vi "email_alert.vi"(6 "Email Alert - Message":string, 9 "Email Alert - Engineer":string, 10 "Email Alert - CC":string, 11 "Email ALert - Attachment":path) -> ()   [LabVIEW 2011]
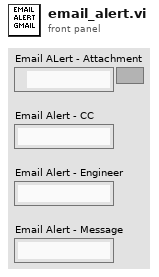
[diagram p1: front panel]
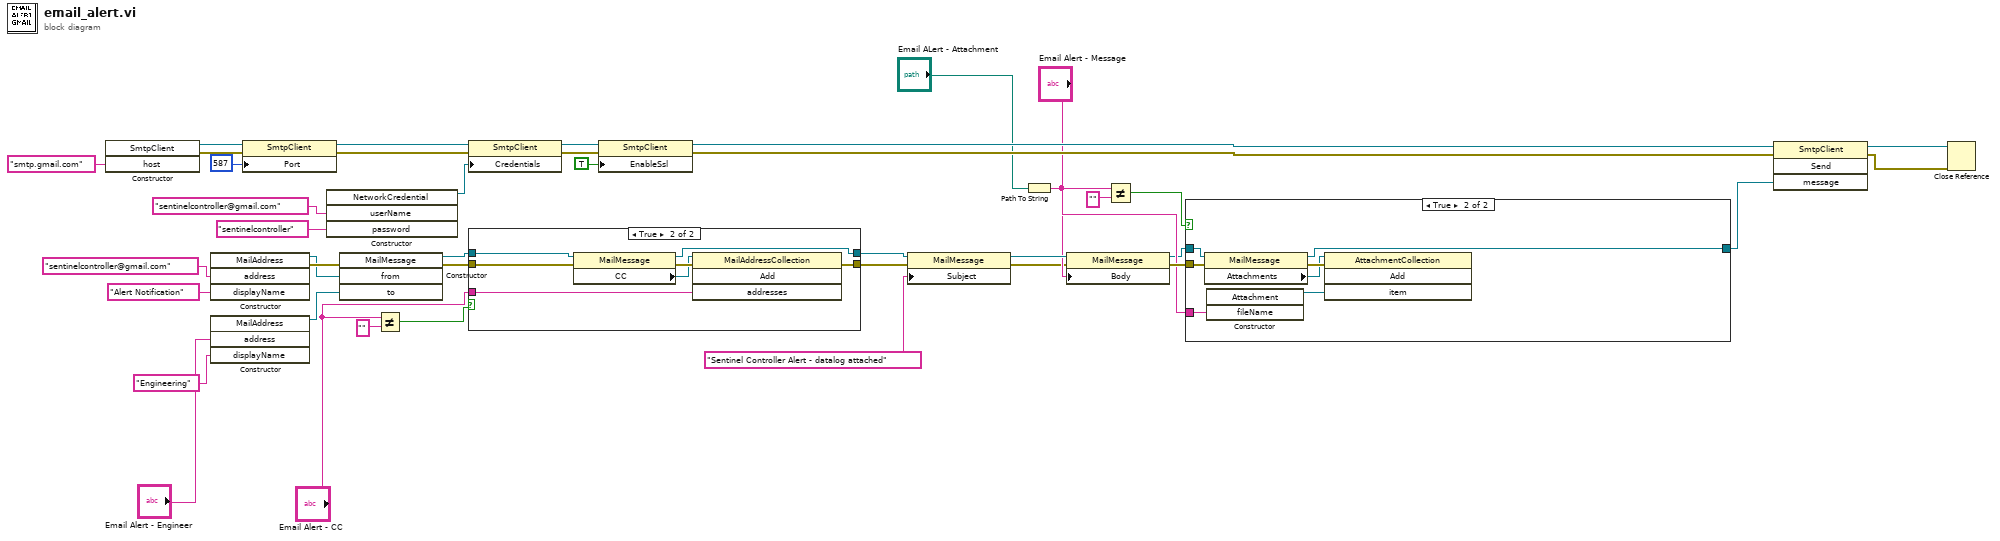
[diagram p0: block diagram]
diagram:
  n1 = constructor class="SmtpClient"("host"="smtp.gmail.com") -> (reference out=w10:refnum<k24>, error out=w13:errorcluster)  [unwired: 3 in, 2 out]
  n2 = constructor class="MailAddress"("address"="sentinelcontroller@gmail.com", "displayName"="Alert Notification") -> (reference out=w4:refnum<k24>, error out=w31:errorcluster)  [unwired: 3 in, 3 out]
  n3 = constructor class="MailAddress"("address"="Email Alert - Engineer", "displayName"="Engineering") -> (reference out=w3:refnum<k24>)  [unwired: 3 in, 4 out]
  n4 = property class="SmtpClient"(reference=w10, error in=w13, "Port"=587) -> (reference out=w11:refnum<k24>, error out=w14:errorcluster)
  n5 = constructor class="NetworkCredential"("userName"="sentinelcontroller@gmail.com", "password"="sentinelcontroller") -> (reference out=w9:refnum<k24>)  [unwired: 3 in, 4 out]
  n6 = constructor class="MailMessage"(error in=w31, "from"=w4, "to"=w3) -> (reference out=w24:refnum<k24>, error out=w25:errorcluster)  [unwired: 2 in, 3 out]
  n7 = Not Equal?(x="Email Alert - CC", y="") -> (x != y?=w22:bool)
  n8 = property class="SmtpClient"(reference=w11, error in=w14, "Credentials"=w9) -> (reference out=w12:refnum<k24>, error out=w15:errorcluster)
  n9 = case shown="True" w22 {
    tunnel: "Email Alert - CC" -> [_ w48]
    tunnel: w24 -> [w43 w47]
    tunnel: w25 -> [w42 w46]
    tunnel: [w43 w45] -> w26
    tunnel: [w42 w44] -> w27
    frame False {
    }
    frame True {
      n10 = property class="MailMessage"(reference=w47, error in=w46) -> (reference out=w45:refnum<k24>, error out=w50:errorcluster, "CC"=w49:refnum<k24>)
      n11 = invoke class="MailAddressCollection" method="Add"(reference=w49, error in=w50, "addresses"=w48) -> (error out=w44:errorcluster)  [unwired: 1 in, 3 out]
    }
  }
  n12 = property class="SmtpClient"(reference=w12, error in=w15, "EnableSsl"=TRUE) -> (reference out=w30:refnum<k24>, error out=w29:errorcluster)
  n13 = property class="MailMessage"(reference=w26, error in=w27, "Subject"="Sentinel Controller Alert - datalog attached") -> (reference out=w8:refnum<k24>, error out=w5:errorcluster)
  n14 = Path To String(path="Email ALert - Attachment") -> (string=w20:string)
  n15 = property class="MailMessage"(reference=w8, error in=w5, "Body"="Email Alert - Message") -> (reference out=w16:refnum<k24>, error out=w32:errorcluster)
  n16 = Not Equal?(x=w20, y="") -> (x != y?=w19:bool)
  n17 = case shown="True" w19 {
    tunnel: w16 -> [w51 w55]
    tunnel: [w51 w54] -> w28
    tunnel: w20 -> [_ w53]
    tunnel: w32 -> [_ w52]
    frame False {
    }
    frame True {
      n18 = property class="MailMessage"(reference=w55, error in=w52) -> (reference out=w54:refnum<k24>, error out=w58:errorcluster, "Attachments"=w56:refnum<k24>)
      n19 = constructor class="Attachment"("fileName"=w53) -> (reference out=w57:refnum<k24>)  [unwired: 3 in, 3 out]
      n20 = invoke class="AttachmentCollection" method="Add"(reference=w56, error in=w58, "item"=w57) -> ()  [unwired: 1 in, 4 out]
    }
  }
  n21 = invoke class="SmtpClient" method="Send"(reference=w30, error in=w29, "message"=w28) -> (reference out=w2:refnum<k24>, error out=w1:errorcluster)  [unwired: 1 in, 2 out]
  n22 = Close Reference(reference=w2, error in (no error)=w1) -> ()  [unwired: 1 out]
